vi "Get Parameter Value - Double.vi"(7 "Default value":dbl, 8 "error in (no error)":errorcluster, 9 "Parameter name":string, 10 "Config name":string, 11 "Config in":refnum<class "Config.lvclass">) -> (0 "error out":errorcluster, 2 "Value":dbl, 3 "Config out":refnum<class "Config.lvclass">)   [LabVIEW 2026, in "TALOS.lvlib" / "Classes.lvlib" / "Config.lvclass"]
doc: "Get the parameter's value (double) from the specified configuration"
uses:
  Config.lvclass
  Ancestor/Ancestor/Ancestor.lvclass/Ancestor.ctl
  FGV/Error Memory/Get Error Description.vi
  Support VIs/Get PC name.vi
  Ancestor/Ancestor/Read ID.vi
  Support VIs/Get Class Name.vi
  <vilib>/Utility/error.llb/Clear Errors.vi
  FGV/Error Memory/Error Memory Core.vi
  <vilib>/AdvancedString/Delimited String to 1D String Array.vi
  <vilib>/AdvancedString/Delimited String to 1D String Array (string).vi
  Support VIs/Circus Root Path.vi
  FGV/Error Memory/Error Crt Lvl checker.vi
  FGV/Error Memory/Error Memory Core.vi/40c8088d-b597-4017-91af-faa98e00292e.vi
  FGV/Error Memory/Error Memory Core.vi/d4a3ab98-063c-4e44-b43d-fbdcfe6c2be2.vi
  Support VIs/Global Memory.vi
  <vilib>/Utility/LVClass/Get LV Class Name.vi
  Support VIs/Is in Packed Library.vi
  Support VIs/TALOS Root path.vi
  Support VIs/Read CSV worksheet.vi
  Support VIs/Global Constants.vi
  <vilib>/Utility/error.llb/General Error Handler.vi
  Support VIs/Error Log.vi
  Ancestor/Ancestor/Ancestor.lvclass
  <vilib>/Comparison/Equal/Equal Functor/Equal Functor.lvclass
  TALOS.lvlib
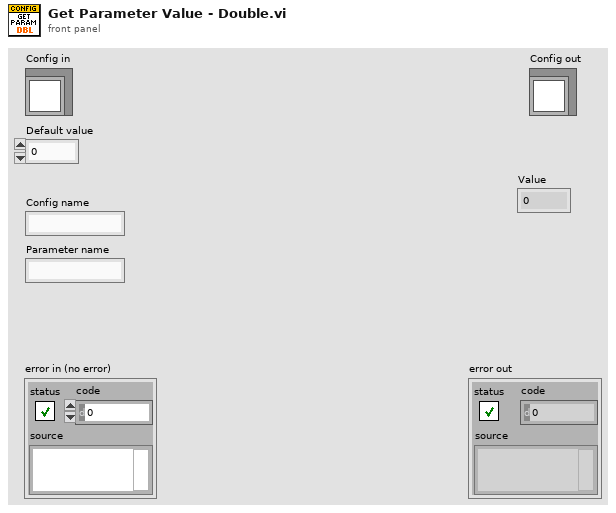
[diagram p1: front panel]
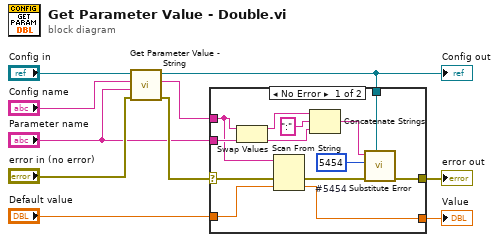
[diagram p0: block diagram]
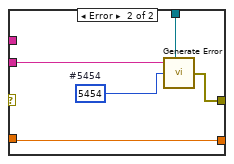
[diagram p2: hidden frame]
diagram:
  n1 = call "Get Parameter Value - String.vi"("error in (no error)"="error in (no error)", "Parameter name"="Parameter name", "Config name"="Config name", "Config in"="Config in") -> ("error out"=w7:errorcluster, "Value"=w1:string, "Config out"=w4:refnum<class "Config.lvclass">)  [unwired: 5 in]
  "Config out" <- w4
  n2 = case shown="No Error" w7 {
    selector: w7 -> [w18 _]
    tunnel: [w19 w24] -> w3
    tunnel: w4 -> [w22 w27]
    tunnel: [w21 w28] -> w2
    tunnel: "Default value" -> [w17 w24]
    tunnel: "Parameter name" -> [w16 w25]
    tunnel: w1 -> [w15 _]
    frame No Error {
      w20 = 5454  # #5454
      n3 = Swap Values(12:w15, 14:w16) -> (1:w13:string, 3:w14:string)  [unwired: 1 in]
      n4 = Scan From String(input string=w15, error in=w18, default 1=w17) -> (error out=w23:errorcluster, output 1=w19:dbl)  [unwired: 2 in, 2 out]
      n5 = Concatenate Strings(w13, ":" ("string"), w14) -> (w11:string)
      n6 = call "Substitute Error.vi"("LabVIEW Object"=w22, "error in (no error)"=w23, "Error Code"=w20, "Optional String"=w11) -> ("error out"=w21:errorcluster)  [unwired: 7 in]
    }
    frame Error {
      w26 = 5454  # #5454
      n7 = call "Generate Error.vi"("Optional String"=w25, "Class"=w27, "Error Code"=w26) -> ("error out"=w28:errorcluster)  [unwired: 4 in]
    }
  }
  "error out" <- w2
  "Value" <- w3
